vi "Get Type Color.vi"(8 "error in (no error)":errorcluster, 11 "Value Editor Base in":refnum<class "Value Editor Base.lvclass">) -> (0 "error out":errorcluster, 2 "Type Color":u32(colorbox), 3 "Value Editor Base out":refnum<class "Value Editor Base.lvclass">)   [LabVIEW 2020, in "Value Editor Base.lvclass"]
uses:
  Value Editor Base.lvclass
  Value Editor Base.lvclass/Value Editor Base.ctl
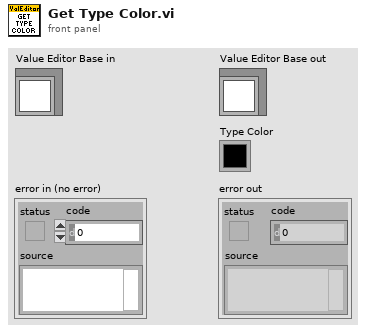
[diagram p1: front panel]
types:
  T1 = typedef "Value Editor Base.lvclass/Ref Data.ctl" = cluster{"Type Descriptor":T2, "Terminal Mode":T6, "Value":variant}
  T2 = typedef "FlexBlocks.lvlib/Type Descriptor.ctl" = cluster{"Name":string, "Direction":T3, "Default":variant, "Min":variant, "Max":variant, "Step":variant, "Value Mode":T4, "Required":bool, "Connpane Index":i32, "Special Terminal":T5, "Color":u32, "Options":string[], "Type String":string, "Sort":i32, "Item Path":path}
  T3 = typedef "FlexBlocks.lvlib/Terminal Direction.ctl" = enum16{"Sink", "Source"}
  T4 = typedef "FlexBlocks.lvlib/Value Mode.ctl" = enum16{"Normal", "Range", "Select"}
  T5 = typedef "FlexBlocks.lvlib/Special Terminal.ctl" = enum16{"None", "Action", "Init", "Tag", "State in", "State out", "Error"}
  T6 = typedef "FlexBlocks.lvlib/Terminal Mode.ctl" = enum16{"Channel", "Config", "Value", "Control Ref"}
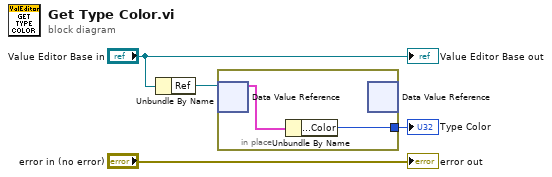
[diagram p0: block diagram]
diagram:
  n1 = Unbundle By Name("Value Editor Base in") -> ("Ref"=w3:refnum<data-value>)
  n2 = in-place {
    in-place-border: [w5] -> w1
    n3 = in-place-dvr #1(w3) -> (w6:T1)  [unwired: 1 out]
    n4 = Unbundle By Name(w6) -> ("Type Descriptor.Color"=w5:u32)
    n5 = in-place-dvr #1() -> ()  [unwired: 1 in, 2 out]
  }
  "Type Color" <- w1
  "error out" <- "error in (no error)"
  "Value Editor Base out" <- "Value Editor Base in"
